vi "init.vi"(8 "error in (no error)":errorcluster, 11 "SystemController in":refnum<class "SystemController.lvclass">) -> (0 "error out":errorcluster, 3 "SystemController out":refnum<class "SystemController.lvclass">)   [LabVIEW 2015, in "SystemController.lvclass"]
uses:
  SystemController/SystemController.lvclass
  Configuration/SystemController.ctl
  SystemController/SystemController.lvclass/SystemController.ctl
  ConfigurationThisComponent/ConfigurationThisComponent.lvclass
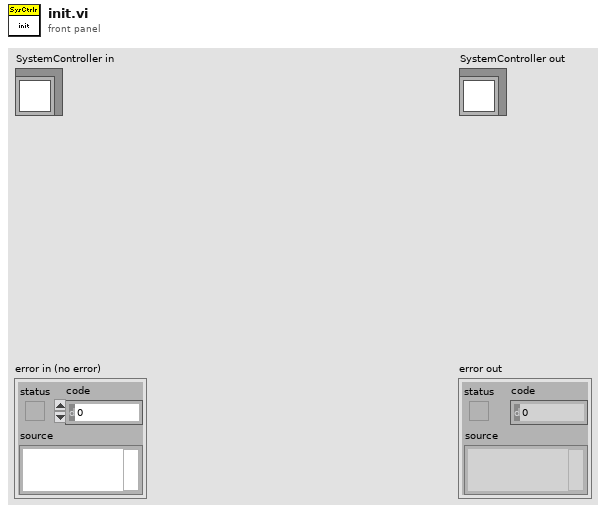
[diagram p1: front panel]
types:
  T1 = typedef "SystemController.ctl" = cluster{"PreconditioningRamp Rate (%/s)":dbl[unit], "Stiffness Test Ramp Rate (%/s)":dbl[unit], "Preconditioning Ramp Target":cluster{"Displacement":dbl[unit]}, "Stiffness Test Ramp Targets":cluster{"Displacement":dbl[unit], "Target Force":dbl[unit]}, "Settling":cluster{"Displacement Max StDev":dbl[unit], "Evaluation Time":dbl[unit]}}
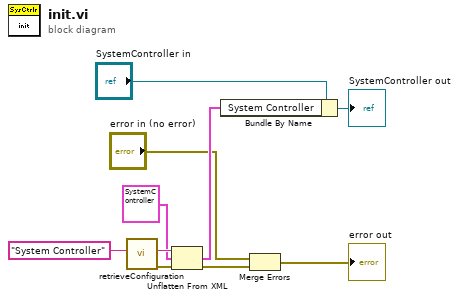
[diagram p0: block diagram]
diagram:
  n1 = call "retrieveConfiguration.vi"("configName"="System Controller") -> ("error out"=w7:errorcluster, "xmlConfig"=w6:string)  [unwired: 8 in, 1 out]
  n2 = Unflatten From XML(xml string=w6, type=T1 {"PreconditioningRamp Rate (%/s)"=2.0, "Stiffness Test Ramp Rate (%/s)"=2.0, "Preconditioning Ramp Target"={"Displacement"=2e-06}, "Stiffness Test Ramp Targets"={"Displacement"=2e-06, "Target Force"=8.896444}, "Settling"={"Displacement Max StDev"=2e-06, "Evaluation Time"=2.0}} ("System Controller"), error in (no error)=w7) -> (value=w10:T1, error out=w9:errorcluster)
  n3 = Bundle By Name(cluster="SystemController in", "System Controller"=w10) -> (→"SystemController out":refnum<class "SystemController.lvclass">)
  n4 = Merge Errors("error in (no error)", w9) -> (→"error out":errorcluster)
